vi "Tester.vi"() -> ()   [LabVIEW 2012]
uses:
  Joystick Event.ctl
panel:
  in  "Slide 2":dbl(slide)=0.25252525252525265 scale=-1.0..1.0
  in  "Slide":dbl(slide)=0.2727272727272728 scale=-1.0..1.0
  out "Outputs":T1={"Slider 1"=0.0, "Slider 2"=-0.007874015748031496}
  in  "Record":bool=TRUE
  in  "Save":bool
  in  "Playback":bool
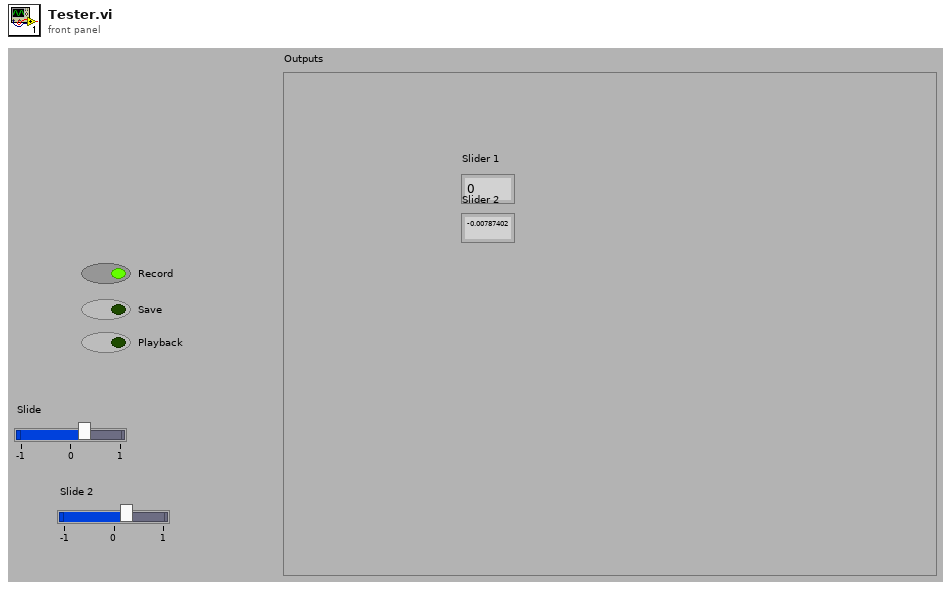
[diagram p1: front panel]
types:
  T1 = typedef "Joystick Event.ctl" = cluster{"Slider 1":dbl, "Slider 2":dbl}
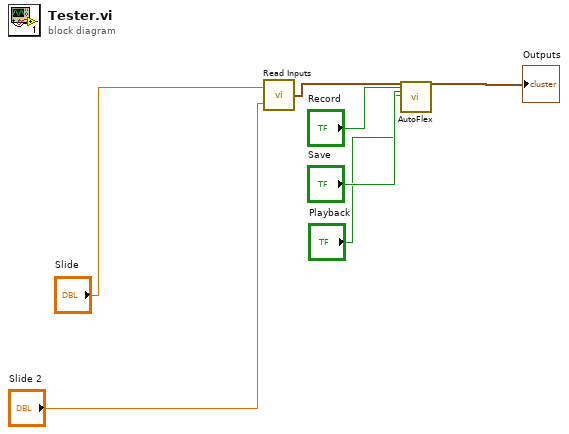
[diagram p0: block diagram]
diagram:
  n1 = call "Read Inputs.vi"("Slider 2"="Slide 2", "Slider 1"="Slide") -> ("Inputs"=w7:cluster{"Slider 1":dbl, "Slider 2":dbl})
  n2 = call "AutoFlex.vi"("Inputs"=w7, "Record"="Record", "Save"="Save", "Playback"="Playback") -> ("Outputs"=→"Outputs":T1)  [unwired: 4 in, 19 out]
